vi "Change Image Source.vi"(8 "error in (no error)":errorcluster, 9 "Image Source Enq":refnum<class "Message Enqueuer.lvclass">, 10 "Image Source":string, 11 "AF IMAQ Display in":refnum<class "HIJ Vision Display.lvclass">) -> (0 "error out":errorcluster, 3 "AF IMAQ Display out":refnum<class "HIJ Vision Display.lvclass">)   [LabVIEW 2014, in "HIJ Vision Display.lvlib" / "HIJ Vision Display.lvclass"]
uses:
  HIJ Vision Display.lvclass
  <vilib>/ActorFramework/Message Enqueuer/Message Enqueuer.lvclass
  HIJ Vision Display.lvclass/HIJ Vision Display.ctl
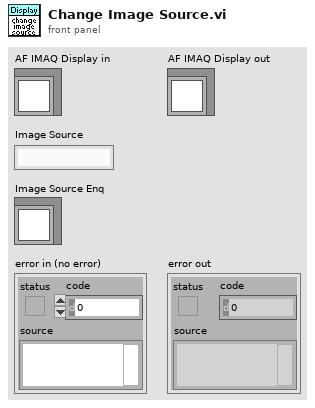
[diagram p1: front panel]
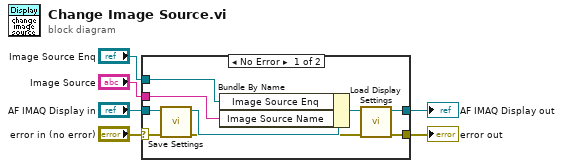
[diagram p0: block diagram]
diagram:
  n1 = case shown="No Error" "error in (no error)" {
    selector: "error in (no error)" -> [w9 w17]
    tunnel: [w8 w17] -> w5
    tunnel: [w13 w16] -> w3
    tunnel: "AF IMAQ Display in" -> [w15 w16]
    tunnel: "Image Source" -> [w11 _]
    tunnel: "Image Source Enq" -> [w7 _]
    frame No Error {
      n2 = call-dynamic "Save Settings.vi"("error in (no error)"=w9, "IMAQ Display in"=w15) -> ("error out"=w10:errorcluster, "IMAQ Display out"=w14:refnum<class "HIJ Vision Display.lvclass">)  [unwired: 8 in]
      n3 = Bundle By Name(cluster=w14, "Image Source Enq"=w7, "Image Source Name"=w11) -> (w12:refnum<class "HIJ Vision Display.lvclass">)
      n4 = call-dynamic "Load Display Settings.vi"("error in (no error)"=w10, "AF IMAQ Display in"=w12) -> ("error out"=w8:errorcluster, "AF IMAQ Display out"=w13:refnum<class "HIJ Vision Display.lvclass">)  [unwired: 8 in]
    }
    frame Error {
    }
  }
  "error out" <- w5
  "AF IMAQ Display out" <- w3
